vi "Loading Eye Picture.vi"(8 "error in (no error)":errorcluster, 10 "名称或相对路径":string, 11 "Image Name":string="untitled") -> (0 "error out":errorcluster, 3 "Image Out":T1)   [LabVIEW 2015, in "Utility VIs.lvlib"]
uses:
  Utility VIs.lvlib
  <vilib>/vision/Image Controls.llb/IMAQ Image.ctl
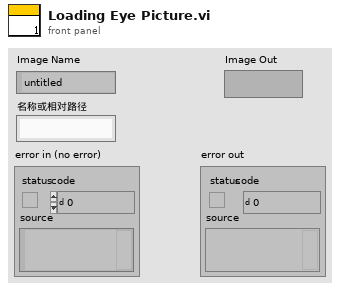
[diagram p1: front panel]
types:
  T1 = typedef "IMAQ Image.ctl" = refnum<image>
  T2 = typedef "Image Type" = u32
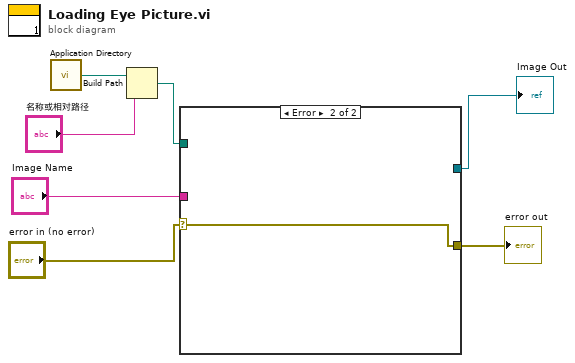
[diagram p0: block diagram]
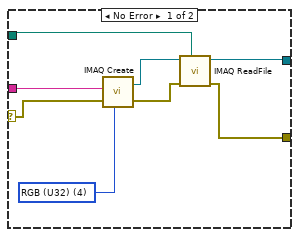
[diagram p2: hidden frame]
diagram:
  n1 = call <vilib>:"Application Directory.vi"() -> ("Application Directory"=w7:path)
  n2 = Build Path(base path=w7, name or relative path="名称或相对路径") -> (appended path=w5:path)
  n3 = case shown="Error" "error in (no error)" {
    selector: "error in (no error)" -> [w8 w16]
    tunnel: w5 -> [w15 _]
    tunnel: "Image Name" -> [w14 _]
    tunnel: [w10 _] -> w3
    tunnel: [w9 w16] -> w2
    frame No Error {
      w11 = T2 4 items=["Grayscale (U8)", "Grayscale (I16)", "Grayscale (SGL)", "Complex (CSG)", "RGB (U32)", "HSL (U32)", "RGB (U64)", "Grayscale (U16)"] ("Image Type")
      n4 = call "IMAQ Create"("Image Name"=w14, "Image Type"=w11, "error in (no error)"=w8) -> ("New Image"=w12:T1, "error out"=w13:errorcluster)  [unwired: 2 in]
      n5 = call "IMAQ ReadFile"("File Path"=w15, "error in (no error)"=w13, "Image"=w12) -> ("error out"=w9:errorcluster, "Image Out"=w10:T1)  [unwired: 4 in, 3 out]
    }
    frame Error {
    }
  }
  "Image Out" <- w3
  "error out" <- w2
